vi "Get Software Limit Configuration.vi"(4 "error in (no error)":errorcluster, 6 "Axis (1)":i32=1 min=1 max=3, 7 "VISA resource name":refnum<visa-resource-name>) -> (0 "error out":errorcluster, 2 "Software limit Configuration":T1, 3 "VISA resource name out":refnum<visa-resource-name>)   [LabVIEW 2012, in "Newport ESP301.lvlib"]
doc: "This command is used to get the software limit checking and event handling for axis specified with <B>Axis (1)</B>.\nNOTE: If bit-0 or both bits-1 and -2 are set to zero(0) then no action will be taken by the controller."
uses:
  Newport ESP301.lvlib
panel:
  # "reserved"
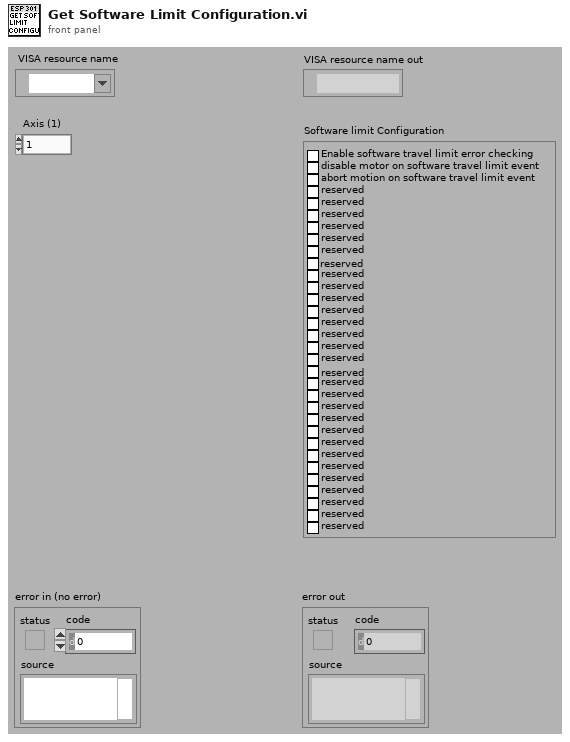
[diagram p1: front panel]
types:
  T1 = cluster{"Enable software travel limit error checking":bool, "disable motor on software travel limit event":bool, "abort motion on software travel limit event":bool, "reserved":bool, "reserved":bool, "reserved  ":bool, "reserved  ":bool, "reserved":bool, "reserved  ":bool, bool, "reserved":bool, "reserved":bool, "reserved ":bool, "reserved ":bool, "reserved":bool, "reserved ":bool, "reserved":bool, "reserved ":bool, "reserved ":bool, "reserved ":bool, "reserved ":bool, "reserved ":bool, "reserved ":bool, "reserved ":bool, "reserved ":bool, "reserved ":bool, "reserved ":bool, "reserved ":bool, "reserved ":bool, "reserved ":bool, "reserved ":bool, "reserved":bool}
  T2 = cluster{"Boolean array[0]":bool, "Boolean array[1]":bool, "Boolean array[2]":bool, "Boolean array[3]":bool, "Boolean array[4]":bool, "Boolean array[5]":bool, "Boolean array[6]":bool, "Boolean array[7]":bool, "Boolean array[8]":bool, "Boolean array[9]":bool, "Boolean array[10]":bool, "Boolean array[11]":bool, "Boolean array[12]":bool, "Boolean array[13]":bool, "Boolean array[14]":bool, "Boolean array[15]":bool, "Boolean array[16]":bool, "Boolean array[17]":bool, "Boolean array[18]":bool, "Boolean array[19]":bool, "Boolean array[20]":bool, "Boolean array[21]":bool, "Boolean array[22]":bool, "Boolean array[23]":bool, "Boolean array[24]":bool, "Boolean array[25]":bool, "Boolean array[26]":bool, "Boolean array[27]":bool, "Boolean array[28]":bool, "Boolean array[29]":bool, "Boolean array[30]":bool, "Boolean array[31]":bool}
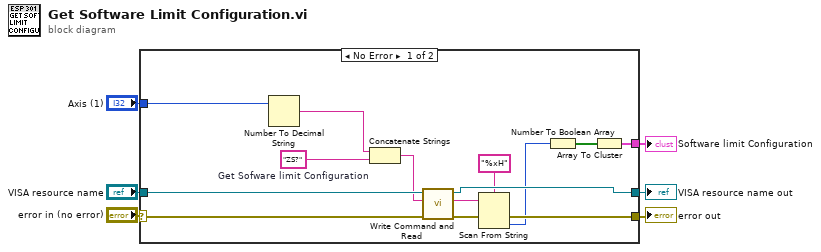
[diagram p0: block diagram]
diagram:
  n1 = case shown="No Error" "error in (no error)" {
    selector: "error in (no error)" -> [w18 w22]
    tunnel: [w10 w22] -> w6
    tunnel: "VISA resource name" -> [w20 w21]
    tunnel: [w19 w21] -> w5
    tunnel: "Axis (1)" -> [w15 _]
    tunnel: [w7 _] -> w1
    frame No Error {
      w17 = "ZS?"  # Get Sofware limit Configuration
      n2 = Number To Decimal String(number=w15) -> (decimal integer string=w14:string)  [unwired: 1 in]
      n3 = Concatenate Strings(w14, w17) -> (w16:string)
      n4 = call "Write Command and Read.vi"("error in (no error)"=w18, "Command"=w16, "VISA resource name"=w20) -> ("error out"=w11:errorcluster, "Returned string"=w9:string, "VISA resource name out"=w19:refnum<visa-resource-name>)  [unwired: 2 in, 2 out]
      n5 = Scan From String(format string="%xH" ("chaîne de format"), input string=w9, error in=w11) -> (error out=w10:errorcluster, output 1=w8:u32)  [unwired: 2 in, 2 out]
      n6 = Number To Boolean Array(number=w8) -> (Boolean array=w13:bool[])
      n7 = Array To Cluster(array=w13) -> (cluster=w7:T2)
    }
    frame Error {
    }
  }
  "error out" <- w6
  "VISA resource name out" <- w5
  "Software limit Configuration" <- w1
